vi "GUI Login Window.vi"(9 "Password?":bool, 10 "Password in":string caption="Senha", 11 "Controller IP Address in":string caption="Endereço IP do controlador do FOFB") -> (1 "Cancelled?":bool, 2 "Password out":string="boo500mev", 3 "Controller IP Address out":string="10.0.5.31")   [LabVIEW 2011, in "User Interface Window VIs.lvlib"]
uses:
  User Interface Window VIs.lvlib
panel:
  in  "Cancel":bool
  in  "OK Button":bool
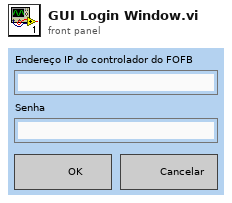
[diagram p1: front panel]
types:
  T1 = enum8{"Enabled", "Disabled", "Disabled and Grayed Out"}
  T2 = typedef "eventvkey.ctl" = enum16{"ASCII", "Enter", "Return", "Shift", "Ctrl", "Alt", "Cmd", "Opt", "Caps", "NumLock", "Clear", "Break", "Up", "Down", "Left", "Right", "Insert", "Delete", "Home", "End", "PageUp", "PageDown", "Escape", "Help", "Pause", "ScrollLock", "F1", "F2", "F3", "F4", "F5", "F6", "F7", "F8", "F9", "F10", "F11", "F12", "F13", "F14", "F15", "F16", "F17", "F18", "F19", "F20", "F21", "F22", "F23", "F24", "Play", "VolumeUp", "VolumeDown", "Mute", "Two Byte Char"}
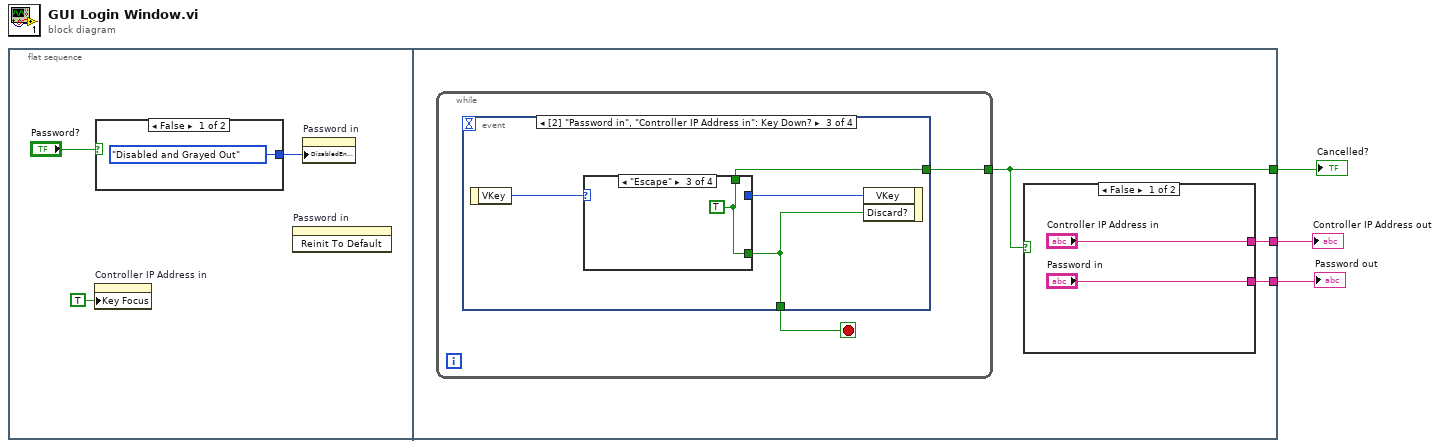
[diagram p0: block diagram]
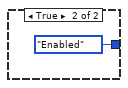
[diagram p2: hidden frame]
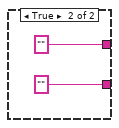
[diagram p3: hidden frame]
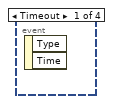
[diagram p4: hidden frame]
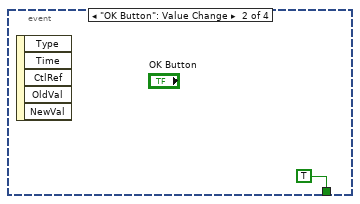
[diagram p5: hidden frame]
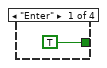
[diagram p6: hidden frame]
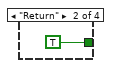
[diagram p7: hidden frame]
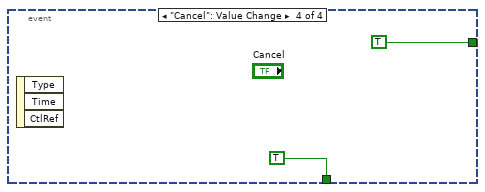
[diagram p9: hidden frame]
diagram:
  n1 = flat-sequence {
    tunnel: [w11] -> w3
    tunnel: [w10] -> w2
    tunnel: [w9] -> w1
    frame #0 {
      n2 = property on="Controller IP Address in" class="Str"("Key Focus"=TRUE) -> ()  [unwired: 2 in, 2 out]
      n3 = case shown="False" "Password?" {
        tunnel: [T1."Disabled and Grayed Out" ("Disabled") T1."Enabled" ("Disabled")] -> w6
        frame False {
        }
        frame True {
        }
      }
      n4 = invoke on="Password in" class="Str" method="Reinit To Default"() -> ()  [unwired: 3 in, 3 out]
      n5 = property on="Password in" class="Str"("DisabledEnum"=w6) -> ()  [unwired: 2 in, 2 out]
    }
    frame #1 {
      n6 = while {
        tunnel: [w17] -> w11
        stop <- w16 stop-if-true
        n7 = event shown="[2] \"Password in\", \"Controller IP Address in\": Key Down?" {
          selector: _ -> [_ _ _ _]
          dyn-events: _ -> [_ _ _ _]
          timeout: _ -> [_ _ _ _]
          tunnel: [_ _ w22 TRUE ("Cancel")] -> w17
          tunnel: [_ TRUE ("Cancel") w19 TRUE ("Cancel")] -> w16
          event Timeout {
            n8 = event-data() -> ()  [unwired: 1 in, 2 out]
          }
          event "OK Button": Value Change {
            n9 = event-data() -> ()  [unwired: 1 in, 5 out]
          }
          event "Password in", "Controller IP Address in": Key Down? {
            n10 = event-data() -> ("VKey"=w21:T2)  [unwired: 1 in]
            n11 = case shown="\"Escape\"" w21 {
              selector: w21 -> [_ _ _ w26]
              tunnel: [TRUE ("Discard?") TRUE ("Discard?") w25 _] -> w19
              tunnel: [_ _ w25 _] -> w22
              tunnel: [_ _ _ w26] -> w20
              frame "Enter" {
              }
              frame "Return" {
              }
              frame "Escape" {
                w25 = TRUE ("Discard?")
              }
              frame "ASCII", Default {
              }
            }
            n12 = event-data("VKey"=w20, "Discard?"=w19) -> ()  [unwired: 1 in, 1 out]
          }
          event "Cancel": Value Change {
            n13 = event-data() -> ()  [unwired: 1 in, 3 out]
          }
        }
      }
      n14 = case shown="False" w11 {
        tunnel: ["Controller IP Address in" "" ("FOFB-Controller IP Address in")] -> w10
        tunnel: ["Password in" "" ("Password in")] -> w9
        frame False {
        }
        frame True {
        }
      }
    }
  }
  "Password out" <- w1
  "Controller IP Address out" <- w2
  "Cancelled?" <- w3
